vi "DigitalOscilloscope[Express].vi"() -> ()   [LabVIEW 2015]
panel:
  out "error out":errorcluster
  in  "Digitizing Paramters":T1
  out "Waveform Graph":dynamicdata(graph)
  in  "stop":bool
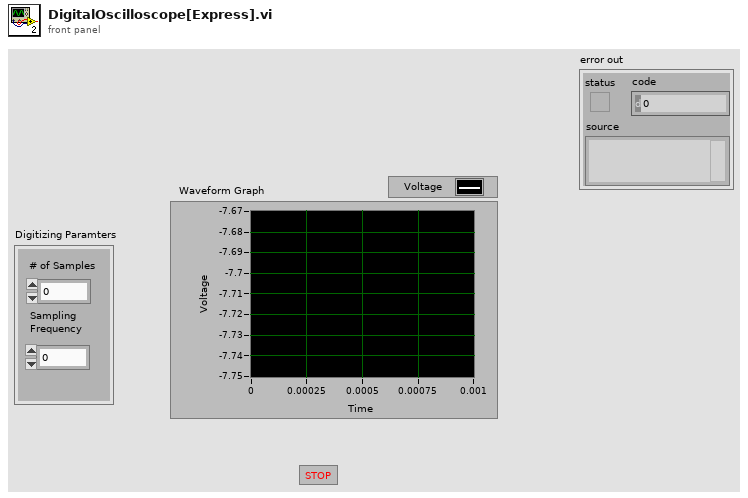
[diagram p1: front panel]
types:
  T1 = cluster{"# of Samples":dbl, "Sampling \nFrequency":dbl}
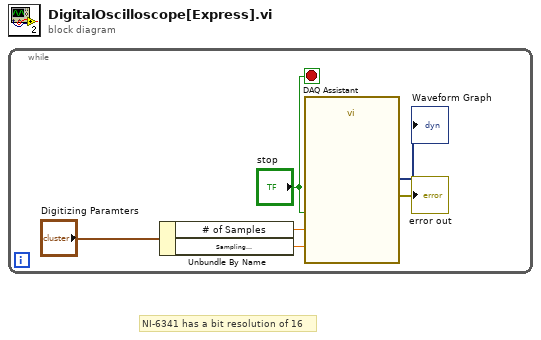
[diagram p0: block diagram]
diagram:
  # "NI-6341 has a bit resolution of 16"
  n1 = while {
    stop <- "stop" stop-if-true
    n2 = Unbundle By Name("Digitizing Paramters") -> ("# of Samples"=w2:dbl, "Sampling \nFrequency"=w1:dbl)
    n3 = call "DAQ Assistant"("rate"=w1, "number of samples"=w2, "stop (T)"="stop") -> ("data"=→"Waveform Graph":dynamicdata, "error out"=→"error out":errorcluster)  [unwired: 14 in, 1 out]
  }
